vi "HTML_Table_Data_datapark_zen42.vi"(8 "entrée d'erreur (pas d'erreur)":errorcluster, 10 "Tableau":string[][](array[string]), 11 "chaîne en entrée":string) -> (0 "sortie d'erreur":errorcluster, 3 "result string":string)   [LabVIEW 2017]
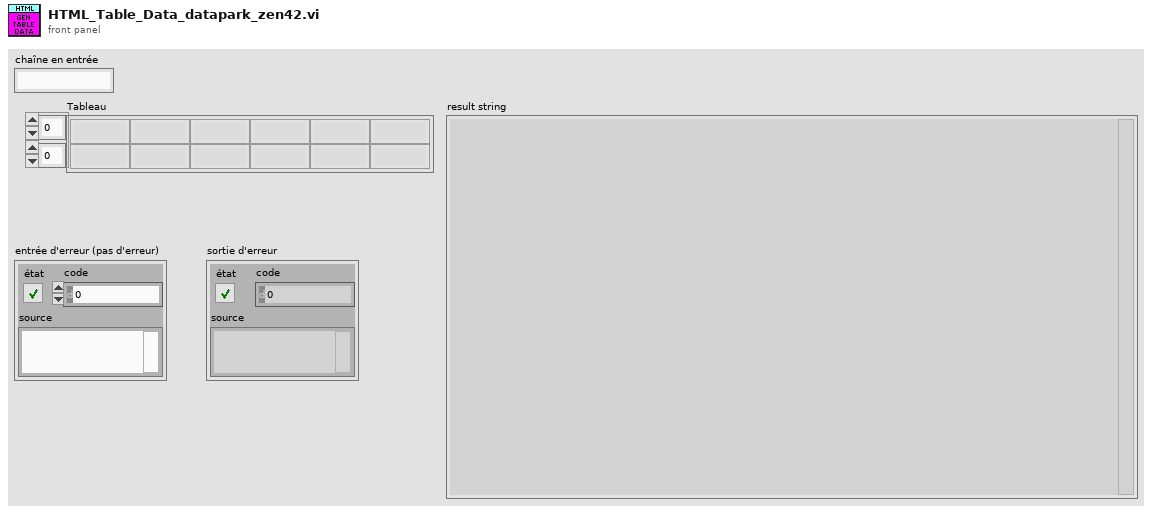
[diagram p1: front panel]
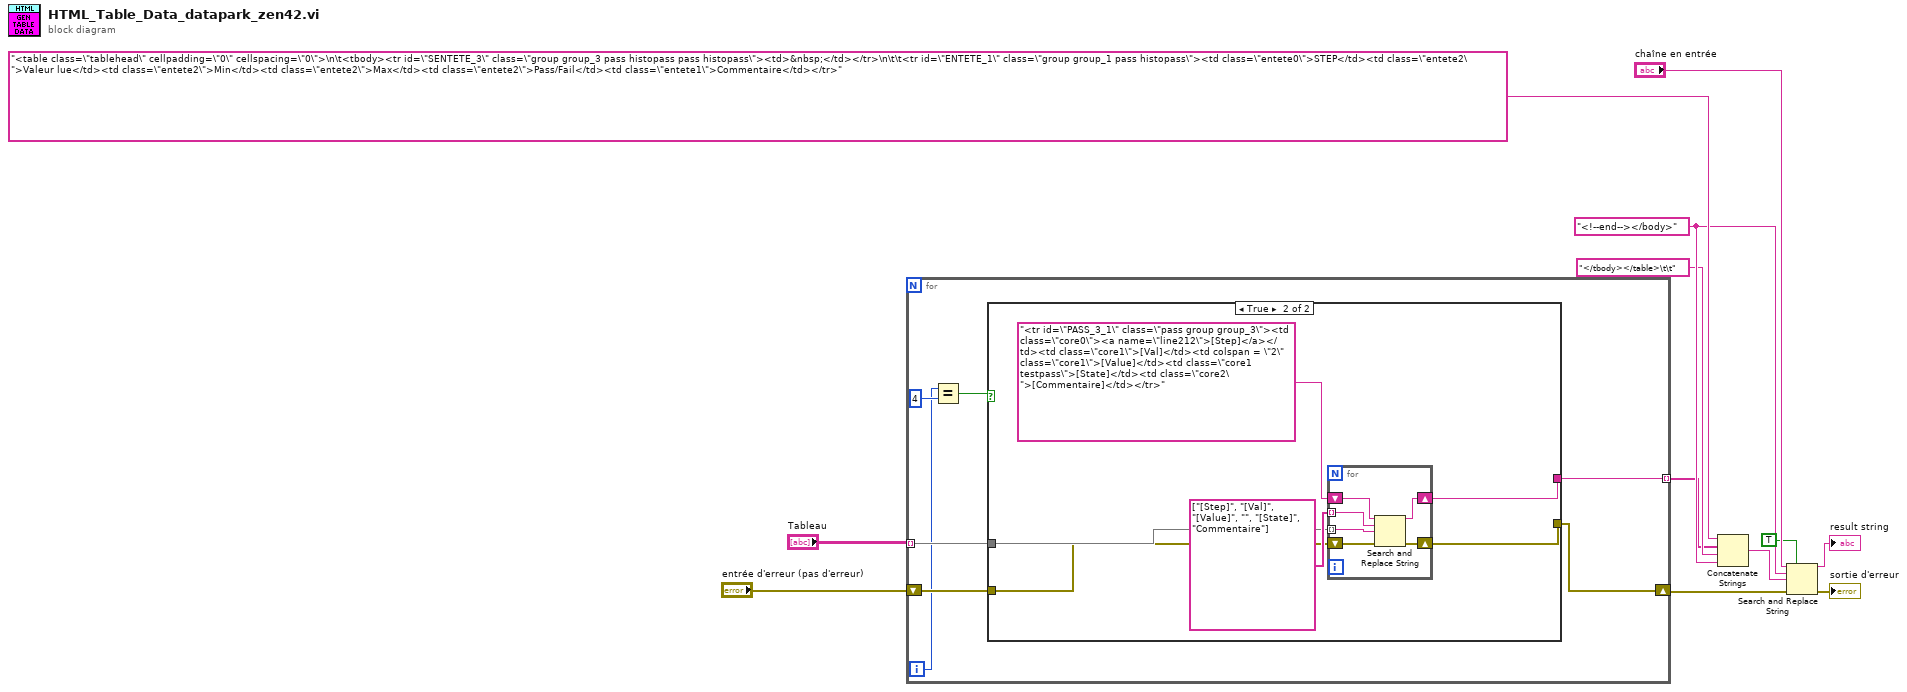
[diagram p0: block diagram]
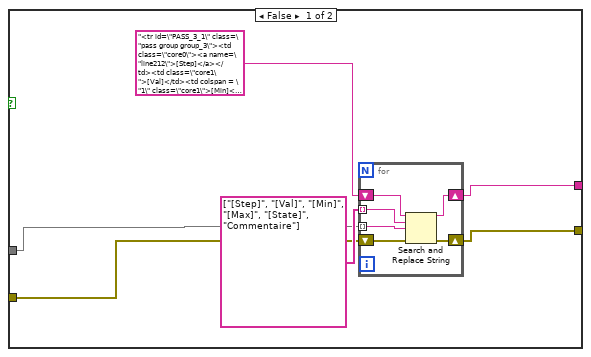
[diagram p2: hidden frame]
diagram:
  w7 = "<!--end--></body>" ("chaîne recherchée")
  n1 = for {
    tunnel: "Tableau" -> [w17] mode=indexing
    tunnel: [w14] -> w1 mode=indexing
    shift-right: [w15] -> w2
    shift-left: "entrée d'erreur (pas d'erreur)" -> [w16]
    i -> [w13]
    n2 = Equal?(x=w13, y=4) -> (x = y?=w19:bool)
    n3 = case shown="True" w19 {
      tunnel: w17 -> [w23 w36]
      tunnel: w16 -> [w22 w35]
      tunnel: [w20 w33] -> w15
      tunnel: [w21 w32] -> w14
      frame False {
        n4 = for {
          tunnel: string[] ["[Step]", "[Val]", "[Min]", "[Max]", "[State]", "Commentaire"] -> [w31] mode=indexing
          tunnel: w23 -> [w30] mode=indexing
          shift-right: [w28] -> w20
          shift-left: w22 -> [w29]
          shift-right: [w26] -> w21
          shift-left: "<tr id=\"PASS_3_1\" class=\"pass group group_3\"><td class=\"core0\"><a name=\"line212\">[Step]</a></td><td class=\"core1\">[Val]</td><td colspan = \"1\" class=\"core1\">[Min]</td><td class=\"core1\">[Max]</td><td class=\"core1 testpass\">[State]</td><td class=\"core2\">[Commentaire]</td></tr>" -> [w27]
          n5 = Search and Replace String(input string=w27, search string=w31, replace string=w30, error in=w29) -> (result string=w26:string, error out=w28:errorcluster)  [unwired: 4 in, 2 out]
        }
      }
      frame True {
        n6 = for {
          tunnel: string[] ["[Step]", "[Val]", "[Value]", "", "[State]", "Commentaire"] -> [w43] mode=indexing
          tunnel: w36 -> [w42] mode=indexing
          shift-right: [w40] -> w33
          shift-left: w35 -> [w41]
          shift-right: [w38] -> w32
          shift-left: "<tr id=\"PASS_3_1\" class=\"pass group group_3\"><td class=\"core0\"><a name=\"line212\">[Step]</a></td><td class=\"core1\">[Val]</td><td colspan = \"2\" class=\"core1\">[Value]</td><td class=\"core1 testpass\">[State]</td><td class=\"core2\">[Commentaire]</td></tr>" -> [w39]
          n7 = Search and Replace String(input string=w39, search string=w43, replace string=w42, error in=w41) -> (result string=w38:string, error out=w40:errorcluster)  [unwired: 4 in, 2 out]
        }
      }
    }
  }
  n8 = Concatenate Strings("<table class=\"tablehead\" cellpadding=\"0\" cellspacing=\"0\">\n\t<tbody><tr id=\"SENTETE_3\" class=\"group group_3 pass histopass pass histopass\"><td>&nbsp;</td></tr>\n\t\t<tr id=\"ENTETE_1\" class=\"group group_1 pass histopass\"><td class=\"entete0\">STEP</td><td class=\"entete2\">Valeur lue</td><td class=\"entete2\">Min</td><td class=\"entete2\">Max</td><td class=\"entete2\">Pass/Fail</td><td class=\"entete1\">Commentaire</td></tr>", w1, "</tbody></table>\t\t", w7) -> (w10:string)
  n9 = Search and Replace String(replace all?=TRUE ("tout remplacer ? (F)"), input string="chaîne en entrée", search string=w7, replace string=w10, error in=w2) -> (result string=→"result string":string, error out=→"sortie d'erreur":errorcluster)  [unwired: 3 in, 2 out]
